vi "MessageProcessingDraft.vi"() -> ()   [LabVIEW 2011]
doc: "Sorts messages in the message log files according to type and extracts how long we were running, how long each mission took, and whether or not the missions were successfully completed. Requires the user to select the message log on startup."
uses:
  Typedefs/missionResults.ctl
panel:
  out "User Messages":string
  out "Mission Results":T1[](array[typedef])
  out "Total time (s)":dbl
  out "Run end":timestamp
  out "Run start":timestamp
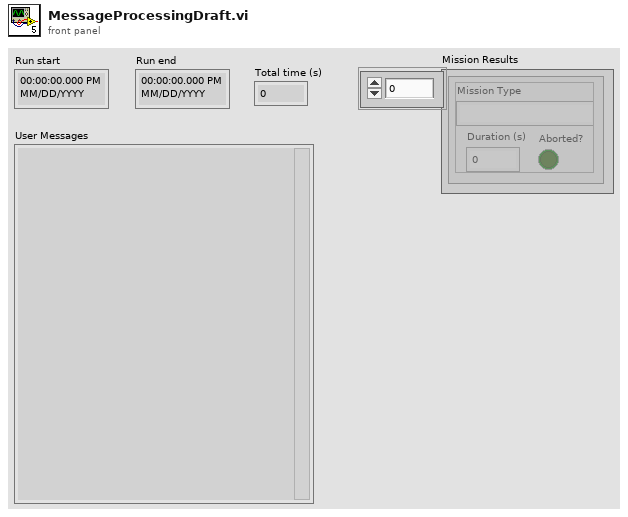
[diagram p1: front panel]
types:
  T1 = typedef "missionResults.ctl" = cluster{"Mission Type":string, "Duration (s)":dbl, "Aborted?":bool}
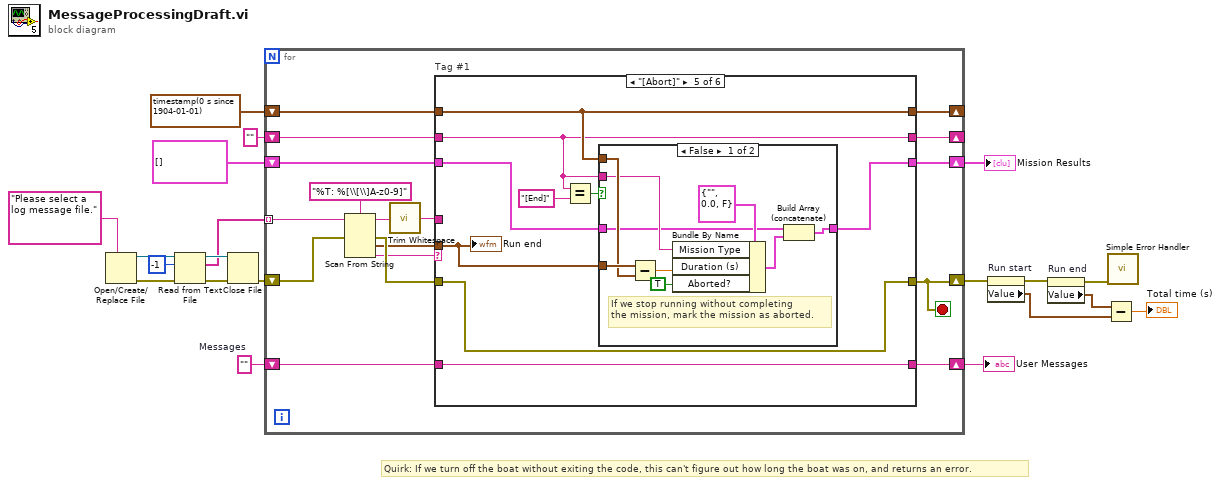
[diagram p0: block diagram]
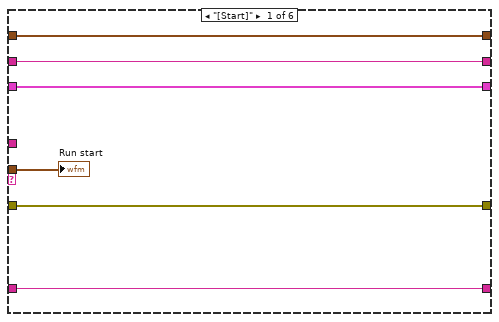
[diagram p2: hidden frame]
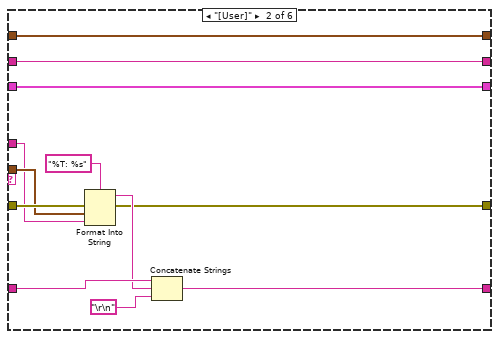
[diagram p3: hidden frame]
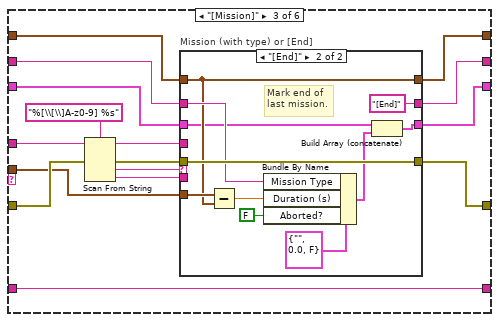
[diagram p4: hidden frame]
diagram:
  w2 = ""  # Messages
  # "Quirk: If we turn off the boat without exiting the code, this can't figure out how long the boat was on, and returns an error."
  n1 = Open/Create/Replace File(prompt="Please select a log message file.") -> (refnum out=w19:refnum<file>, error out=w18:errorcluster)  [unwired: 5 in, 1 out]
  n2 = Read from Text File(file (use dialog)=w19, count=-1, error in=w18) -> (refnum out=w16:refnum<file>, text=w14:string[], error out=w15:errorcluster)  [unwired: 1 in, 1 out]
  n3 = Close File(refnum=w16, error in=w15) -> (error out=w13:errorcluster)  [unwired: 1 out]
  n4 = for {
    tunnel: w14 -> [w37] mode=indexing
    shift-right: [w32] -> w12
    shift-left: w13 -> [w36]
    shift-right: [w24] -> w3
    shift-left: T1[] [] ("Mission Results") -> [w28]
    shift-right: [w26] -> _
    shift-left: timestamp(0 s since 1904-01-01) ("output 1") -> [w27]
    shift-right: [w23] -> _
    shift-left: "" ("remaining string") -> [w25]
    shift-right: [w21] -> w1
    shift-left: w2 -> [w22]
    stop <- w32 stop-if-true
    n5 = Scan From String(format string="%T: %[\\[\\]A-z0-9]", input string=w37, error in=w36) -> (remaining string=w30:string, error out=w34:errorcluster, output 1=w33:timestamp, output 2=w31:string)  [unwired: 3 in, 1 out]
    n6 = call <vilib>:"Trim Whitespace.vi"("string"=w30) -> ("trimmed string"=w29:string)  [unwired: 1 in]
    n7 = case "Tag #1" shown="\"[Abort]\"" w31 {
      tunnel: w34 -> [w42 w50 w69 w91 w95 w115]
      tunnel: [w42 w45 w66 w91 w95 w115] -> w32
      tunnel: w33 -> [w43 w48 w63 _ w96 _]
      tunnel: w29 -> [_ w44 w71 _ _ _]
      tunnel: w28 -> [w39 w53 w60 w88 w98 w112]
      tunnel: w27 -> [w41 w55 w62 w90 w94 w114]
      tunnel: [w41 w55 w61 w90 w94 w114] -> w26
      tunnel: w25 -> [w40 w54 w59 w89 w93 w113]
      tunnel: [w39 w53 w58 w88 w97 w112] -> w24
      tunnel: [w40 w54 w57 w89 w93 w113] -> w23
      tunnel: w22 -> [w38 w52 w56 w87 w92 w111]
      tunnel: [w38 w46 w56 w87 w92 w111] -> w21
      frame "[Start]" {
        "Run start" <- w43
      }
      frame "[User]" {
        n8 = Format Into String(format string="%T: %s", error in=w50, w48, w44) -> (resulting string=w47:string, error out=w45:errorcluster)  [unwired: 1 in]
        n9 = Concatenate Strings(w52, w47, "\r\n") -> (w46:string)
      }
      frame "[Mission]" {
        n10 = Scan From String(format string="%[\\[\\]A-z0-9] %s", input string=w71, error in=w69) -> (remaining string=w64:string, error out=w67:errorcluster, output 1=w68:string, output 2=w65:string)  [unwired: 3 in, 1 out]
        n11 = case "Mission (with type) or [End]" shown="\"[End]\"" w68 {
          selector: w68 -> [w72 _]
          tunnel: w67 -> [w75 w85]
          tunnel: [w75 w85] -> w66
          tunnel: w65 -> [_ _]
          tunnel: w64 -> [_ _]
          tunnel: w63 -> [w74 w82]
          tunnel: w62 -> [_ w81]
          tunnel: [w74 w81] -> w61
          tunnel: w60 -> [w73 w79]
          tunnel: w59 -> [_ w84]
          tunnel: [w73 w77] -> w58
          tunnel: [w72 "[End]"] -> w57
          frame Default {
          }
          frame "[End]" {
            # "Mark end of\nlast mission."
            n12 = Subtract(x=w82, y=w81) -> (x-y=w80:dbl)
            n13 = Bundle By Name(cluster=T1 {"Mission Type"="", "Duration (s)"=0.0, "Aborted?"=FALSE} ("Cluster"), "Mission Type"=w84, "Duration (s)"=w80, "Aborted?"=FALSE) -> (w78:T1)
            n14 = Build Array (concatenate)(w79, w78) -> (w77:T1[])
          }
        }
      }
      frame "[Waypoint]" {
      }
      frame "[Abort]" {
        n15 = Equal?(x=w93, y="[End]") -> (x = y?=w100:bool)
        n16 = case shown="False" w100 {
          tunnel: w93 -> [w104 _]
          tunnel: w98 -> [w103 w110]
          tunnel: [w101 w110] -> w97
          tunnel: w96 -> [w106 _]
          tunnel: w94 -> [w105 _]
          frame False {
            # "If we stop running without completing\nthe mission, mark the mission as aborted."
            n17 = Subtract(x=w106, y=w105) -> (x-y=w107:dbl)
            n18 = Bundle By Name(cluster=T1 {"Mission Type"="", "Duration (s)"=0.0, "Aborted?"=FALSE} ("Cluster"), "Mission Type"=w104, "Duration (s)"=w107, "Aborted?"=TRUE) -> (w102:T1)
            n19 = Build Array (concatenate)(w103, w102) -> (w101:T1[])
          }
          frame True {
          }
        }
        "Run end" <- w96
      }
      frame Default {
      }
    }
  }
  "Mission Results" <- w3
  "User Messages" <- w1
  n20 = property on="Run start" class="AbsTime (strict)"(error in=w12) -> (error out=w11:errorcluster, "Value"=w8:timestamp)  [unwired: 1 in, 1 out]
  n21 = property on="Run end" class="AbsTime (strict)"(error in=w11) -> (error out=w10:errorcluster, "Value"=w9:timestamp)  [unwired: 1 in, 1 out]
  n22 = Subtract(x=w9, y=w8) -> (x-y=→"Total time (s)":dbl)
  n23 = call <vilib>:"Simple Error Handler.vi"("error in (no error)"=w10) -> ()  [unwired: 4 in, 5 out]
